vi "Build Context Menu.vi"(8 "error in (no error)":errorcluster, 10 "MenuRef":refnum<k9>, 11 "HIJ Vision Display in":refnum<class "HIJ Vision Display.lvclass">) -> (0 "error out":errorcluster, 2 "MenuRef out":refnum<k9>, 3 "HIJ Vision Display out":refnum<class "HIJ Vision Display.lvclass">)   [LabVIEW 2014, in "HIJ Vision Display.lvlib" / "HIJ Vision Display.lvclass"]
uses:
  HIJ Vision Display.lvclass
  HIJ Vision Display.lvclass/HIJ Vision Display.ctl
  Results and Overlays/Results Base/Analyze Results Base.lvclass
  Results and Overlays/Results Base/Analyze Results Base.lvclass/Analyze Results Base.ctl
  Results and Overlays/Results Base/Read Overlay_.vi
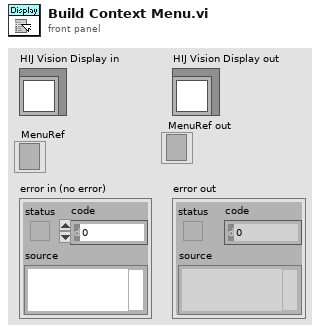
[diagram p1: front panel]
types:
  T1 = typedef "HIJ Vision Display.lvlib/HIJ Vision Display.lvclass/Named ROI.ctl" = cluster{"ROI":cluster{"Global Rectangle":i32[], "Contours":cluster{"Contour Type":u32, "ROI Type":u32, "Points":i32[]}[]}, "Name":string}
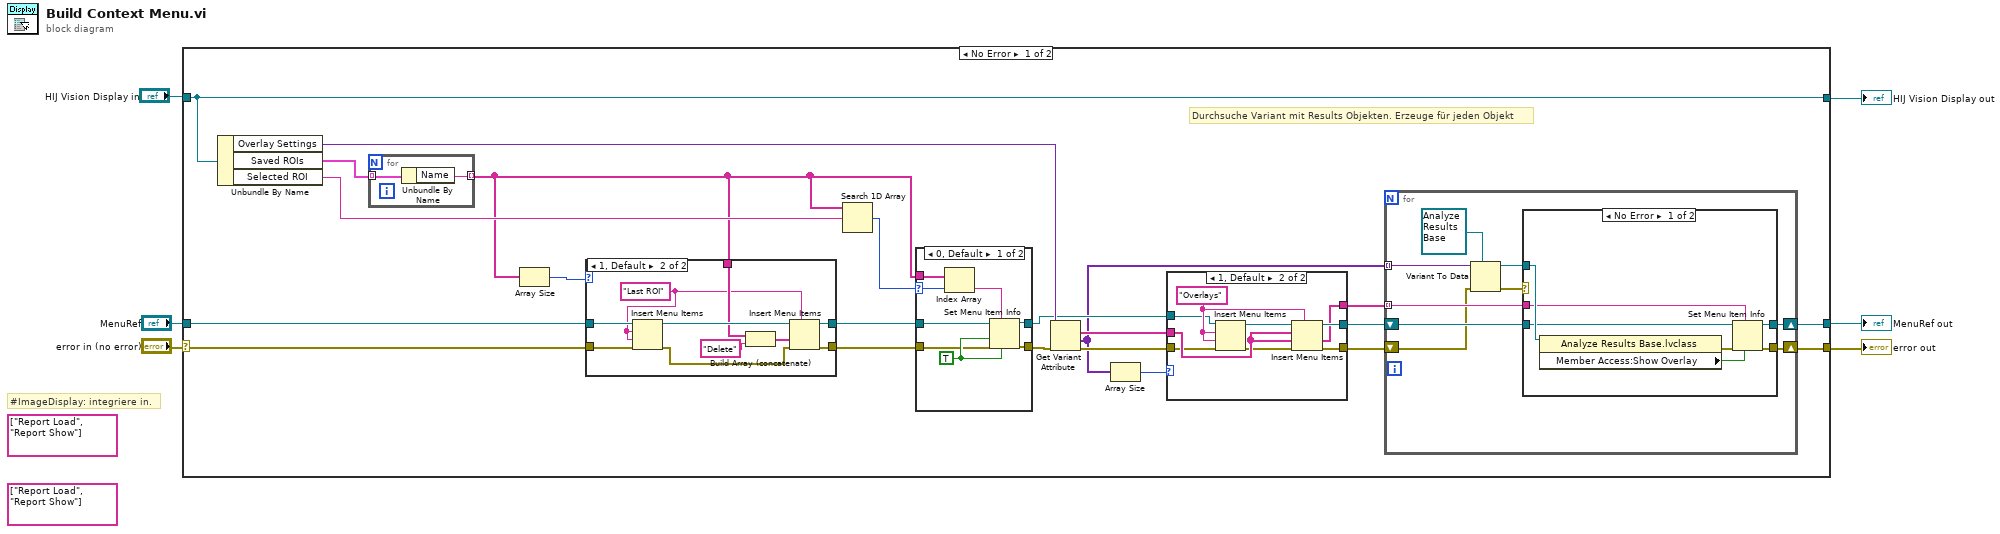
[diagram p0: block diagram]
diagram:
  (unwired) string[] ["Report Load", "Report Show"] ("item names")
  (unwired) string[] ["Report Load", "Report Show"] ("item names")
  # "#ImageDisplay: integriere in."
  n1 = case shown="No Error" "error in (no error)" {
    selector: "error in (no error)" -> [w22 w85]
    tunnel: [w28 w84] -> w4
    tunnel: "HIJ Vision Display in" -> [w28 w84]
    tunnel: "MenuRef" -> [w19 w83]
    tunnel: [w11 w85] -> w2
    tunnel: [w13 w83] -> w1
    frame No Error {
      # "Durchsuche Variant mit Results Objekten. Erzeuge für jeden Objekt"
      n2 = Unbundle By Name(w28) -> ("Overlay Settings"=w18:variant, "Saved ROIs"=w27:T1[], "Selected ROI"=w26:string)
      n3 = for {
        tunnel: w27 -> [w82] mode=indexing
        tunnel: [w81] -> w25 mode=indexing
        n4 = Unbundle By Name(w82) -> ("Name"=w81:string)
      }
      n5 = Array Size(array=w25) -> (size(s)=w24:i32)
      n6 = case shown="1, Default" w24 {
        tunnel: w19 -> [w70 w79]
        tunnel: w25 -> [_ w76]
        tunnel: [w70 w75] -> w20
        tunnel: [w69 w74] -> w21
        tunnel: w22 -> [w69 w71]
        frame 0 {
        }
        frame 1, Default {
          w72 = "Last ROI" ("menu tag")
          n7 = Insert Menu Items(6:w71, 7:w72, 8:w72, 9:w79) -> (0:w80:errorcluster, 3:w78:refnum<k9>)  [unwired: 2 in, 1 out]
          n8 = Build Array (concatenate)(w76, "Delete" ("item names")) -> (w73:string[])
          n9 = Insert Menu Items(5:w72, 6:w80, 7:w73, 9:w78) -> (0:w74:errorcluster, 3:w75:refnum<k9>)  [unwired: 2 in, 1 out]
        }
      }
      n10 = Search 1D Array(1D array=w25, element=w26) -> (index of element=w23:i32)  [unwired: 1 in]
      n11 = case shown="0, Default" w23 {
        selector: w23 -> [w65 _]
        tunnel: w25 -> [w64 _]
        tunnel: w20 -> [w66 w67]
        tunnel: w21 -> [w61 w68]
        tunnel: [w60 w68] -> w16
        tunnel: [w59 w67] -> w10
        frame 0, Default {
          w62 = TRUE ("checked")
          n12 = Index Array(array=w64, index=w65) -> (element=w63:string)
          n13 = Set Menu Item Info(6:w62, 7:w63, 8:w61, 9:w62, 11:w66) -> (0:w60:errorcluster, 3:w59:refnum<k9>)  [unwired: 2 in]
        }
        frame -1 {
        }
      }
      n14 = Get Variant Attribute(Variant=w18, error in=w16) -> (names=w17:string[], values=w8:variant[], error out=w9:errorcluster)  [unwired: 2 in, 1 out]
      n15 = Array Size(array=w8) -> (size(s)=w7:i32)
      n16 = case shown="1, Default" w7 {
        tunnel: w17 -> [w31 w40]
        tunnel: [w30 w39] -> w15
        tunnel: [w29 w38] -> w14
        tunnel: [w31 w37] -> w12
        tunnel: w10 -> [w29 w35]
        tunnel: w9 -> [w30 w33]
        frame 0 {
        }
        frame 1, Default {
          w36 = "Overlays" ("menu tag")
          n17 = Insert Menu Items(6:w33, 7:w36, 8:w36, 9:w35) -> (0:w32:errorcluster, 3:w34:refnum<k9>)  [unwired: 2 in, 1 out]
          n18 = Insert Menu Items(5:w36, 6:w32, 7:w40, 8:w40, 9:w34) -> (0:w39:errorcluster, 1:w37:string[], 3:w38:refnum<k9>)  [unwired: 1 in]
        }
      }
      n19 = for {
        tunnel: w12 -> [w45] mode=indexing
        shift-right: [w44] -> w11
        shift-left: w15 -> [w42]
        shift-right: [w46] -> w13
        shift-left: w14 -> [w47]
        tunnel: w8 -> [w43] mode=indexing
        n20 = Variant To Data(error in=w42, type=refnum<class "Analyze Results Base.lvclass"> refnum ("Analyze Results Base.lvclass"), Variant=w43) -> (data=w48:refnum<class "Analyze Results Base.lvclass">, error out=w41:errorcluster)
        n21 = case shown="No Error" w41 {
          selector: w41 -> [_ w58]
          tunnel: w48 -> [w56 _]
          tunnel: w47 -> [w55 w57]
          tunnel: [w54 w57] -> w46
          tunnel: w45 -> [w53 _]
          tunnel: [w50 w58] -> w44
          frame No Error {
            n22 = property class="Analyze Results Base.lvclass"(reference=w56) -> (error out=w51:errorcluster, "Member Access:Show Overlay"=w52:bool)  [unwired: 1 in, 1 out]
            n23 = Set Menu Item Info(6:w52, 7:w53, 8:w51, 11:w55) -> (0:w50:errorcluster, 3:w54:refnum<k9>)  [unwired: 3 in]
          }
          frame Error {
          }
        }
      }
    }
    frame Error {
    }
  }
  "error out" <- w2
  "HIJ Vision Display out" <- w4
  "MenuRef out" <- w1
